vi "non-HT Subcarrier Mapper.vi"(10 "frequency offset index":fxp<+/-,9,9>) -> (2 "subcarrier valid":bool, 3 "pilot subcarrier":bool)   [LabVIEW 2020]
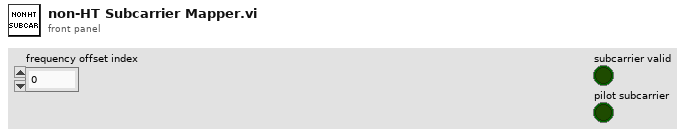
[diagram p1: front panel]
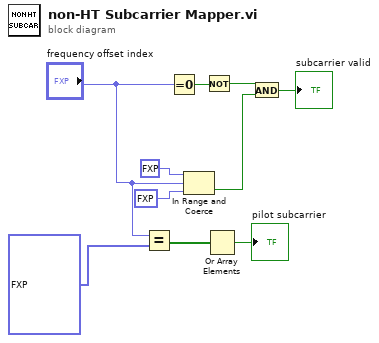
[diagram p0: block diagram]
diagram:
  n1 = Equal?(x="frequency offset index", y=fxp<+/-,9,9>[] [-21.0, -7.0, 7.0, 21.0] ("frequency offset index")) -> (x = y?=w3:bool[])
  n2 = Equal To 0?(x="frequency offset index") -> (x = 0?=w10:bool)
  n3 = In Range and Coerce(upper limit=fxp<+/-,9,9> 27.0, x="frequency offset index", lower limit=fxp<+/-,9,9> -26.0) -> (In Range?=w5:bool)  [unwired: 1 out]
  n4 = Not(x=w10) -> (.not. x?=w9:bool)
  n5 = Or Array Elements(Boolean array=w3) -> (logical OR=→"pilot subcarrier":bool)
  n6 = And(x=w9, y=w5) -> (x .and. y?=→"subcarrier valid":bool)
